vi "FRCts20_WebMethods_ReadData_Competition.vi"(7 "Competition in":T1, 8 "error in (no error)":errorcluster, 11 "httpRequestID":u32) -> (0 "error out":errorcluster, 2 "Competition out":T1, 3 "httpRequestID out":u32)   [LabVIEW 2013, in "FRCts20_WebMethods.lvlib"]
uses:
  Backend/source/VI Source/FRCts20_Backend_API/FRCts20_Backend_API_Competition.ctl
  FRCts20_WebMethods.lvlib
  <vilib>/wsapi/NI_WebServices.lvlib
  Backend/source/VI Source/FRCts20_Backend_API/FRCts20_Backend_API.lvlib
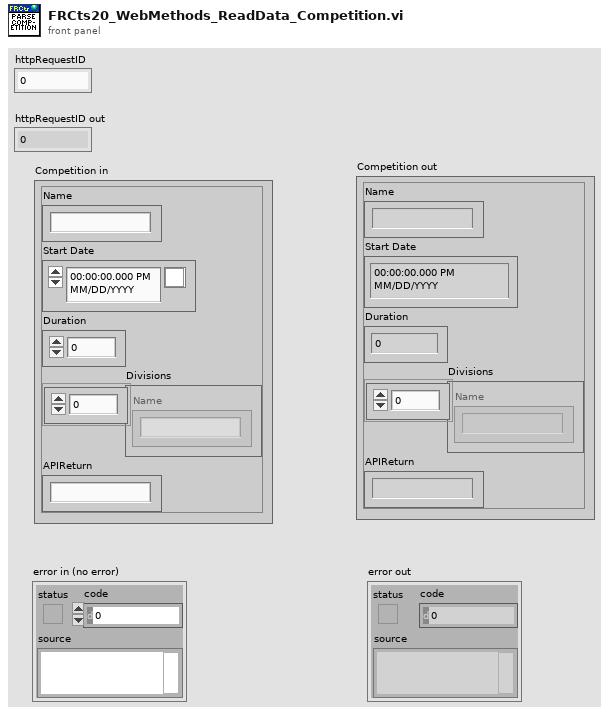
[diagram p1: front panel]
types:
  T1 = typedef "FRCts20_Backend_API.lvlib/FRCts20_Backend_API_Competition.ctl" = cluster{"Name":string, "Start Date":timestamp, "Duration":u8, "Divisions":string[], "APIReturn":string}
  T2 = typedef "FRCts20_WebMethods.lvlib/FRCts20_WebMethods_ctl_returntype.ctl" = string
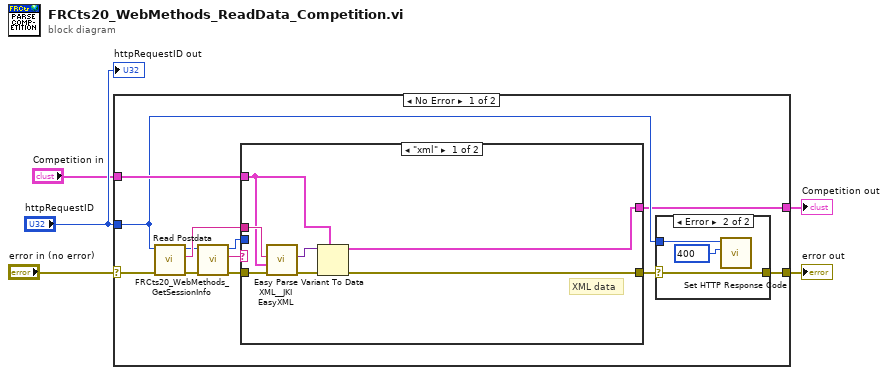
[diagram p0: block diagram]
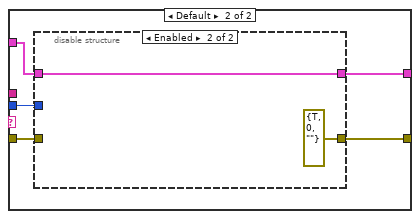
[diagram p3: hidden frame]
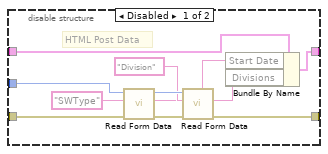
[diagram p4: hidden frame]
diagram:
  n1 = case shown="No Error" "error in (no error)" {
    selector: "error in (no error)" -> [w17 w48]
    tunnel: "httpRequestID" -> [w12 _]
    tunnel: "Competition in" -> [w15 w47]
    tunnel: [w13 w48] -> w4
    tunnel: [w11 w47] -> w1
    frame No Error {
      n2 = call <vilib>:"Read Postdata.vi"("error in (no error)"=w17, "httpRequestID"=w12) -> ("error out"=w9:errorcluster, "postdata"=w16:string, "httpRequestID out"=w8:u32)  [unwired: 7 in]
      n3 = call "FRCts20_WebMethods_GetSessionInfo.vi"("error in"=w9, "httpRequestID"=w8) -> ("error out"=w10:errorcluster, "Return Type"=w6:T2, "httpRequestID out"=w7:u32)  [unwired: 7 in]
      n4 = case shown="\"xml\"" w6 {
        tunnel: w10 -> [w28 w33]
        tunnel: w7 -> [_ w32]
        tunnel: w16 -> [w27 _]
        tunnel: w15 -> [w24 w30]
        tunnel: [w22 w29] -> w14
        tunnel: [w23 w31] -> w11
        frame "xml" {
          # "XML data"
          n5 = call <vilib>:"Easy Parse XML__JKI EasyXML.vi"("error in (no error)"=w28, "LabVIEW Data (Type)"=w24, "XML String"=w27) -> ("error out"=w26:errorcluster, "LabVIEW Data"=w25:variant)  [unwired: 7 in]
          n6 = Variant To Data(error in=w26, type=w24, Variant=w25) -> (data=w23:T1, error out=w22:errorcluster)
        }
        frame Default {
          n7 = disable-structure shown="Enabled" {
            disable-tunnel: w33 -> [w44 _]
            disable-tunnel: w32 -> [w43 _]
            disable-tunnel: [w42 w46] -> w31
            disable-tunnel: w30 -> [w41 w46]
            disable-tunnel: [w39 errorcluster {"status"=TRUE, "code"=0, "source"=""} ("error out")] -> w29
            frame Disabled {
              # "HTML Post Data"
              n8 = call <vilib>:"Read Form Data.vi"("error in (no error)"=w44, "key"="SWType", "httpRequestID"=w43) -> ("error out"=w40:errorcluster, "value"=w34:string, "httpRequestID out"=w37:u32)  [unwired: 5 in, 1 out]
              n9 = call <vilib>:"Read Form Data.vi"("error in (no error)"=w40, "key"="Division", "httpRequestID"=w37) -> ("error out"=w39:errorcluster, "value"=w38:string)  [unwired: 5 in, 2 out]
              n10 = Bundle By Name(cluster=w41, "Start Date"=w34, "Divisions"=w38) -> (w42:T1)
            }
            frame Enabled {
            }
          }
        }
      }
      n11 = case shown="Error" w14 {
        selector: w14 -> [w18 w19]
        tunnel: [w18 w19] -> w13
        tunnel: w12 -> [_ w21]
        frame No Error {
        }
        frame Error {
          w20 = 400 items=["100"=100, "101"=101, "200"=200, "201"=201, "202"=202, "203"=203, "204"=204, "205"=205, "206"=206, "300"=300, "301"=301, "302"=302, "303"=303, "304"=304, "305"=305, "306"=306, "307"=307, "400"=400, "401"=401, "402"=402, "403"=403, "404"=404, "405"=405, "406"=406, "407"=407, "408"=408, "409"=409, "410"=410, "411"=411, "412"=412, "413"=413, "414"=414, "415"=415, "416"=416, "417"=417, "500"=500, "501"=501, "502"=502, "503"=503, "504"=504, "505"=505] ("response code (200)")
          n12 = call <vilib>:"Set HTTP Response Code.vi"("response code (200)"=w20, "httpRequestID"=w21) -> ()  [unwired: 8 in, 2 out]
        }
      }
    }
    frame Error {
    }
  }
  "error out" <- w4
  "Competition out" <- w1
  "httpRequestID out" <- "httpRequestID"
